vi "Check Rectangles Changed.vi"(8 "error in (no error)":errorcluster, 10 "New Tool":refnum<class "Tool Data.lvclass">, 11 "Tool Data in":refnum<class "Tool Data.lvclass">) -> (0 "error out":errorcluster, 2 "Changed":cluster{bool, "index of element":i32}[](array[cluster]), 3 "Tool Data out":refnum<class "Tool Data.lvclass">)   [LabVIEW 2019, in "Tool Data.lvclass"]
uses:
  Tool Data.lvclass
  Typedefs/Tool Data.Check Changes.ctl
  Parse/Rectangle/Rectangle.lvclass
  Parse/CSSProperties/CSSProperties.lvclass
  Parse/Transform.Matrix/Transform.Matrix.lvclass
  Settings/Rectangle Settings/Rectangle Settings.lvclass
  C:/Users/Albro/Documents/GitHub/AFM-Lithography/lvsrc/Classes/Settings/ObjectSettings/ObjectSettings.lvclass
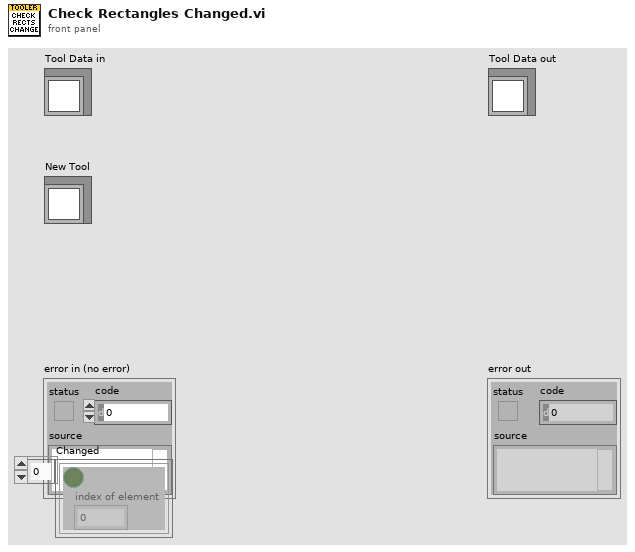
[diagram p1: front panel]
types:
  T1 = typedef "Tool Data.Check Changes.ctl" = cluster{"Data":variant[], "Settings":variant[], "Names":string[]}
  T2 = typedef "Setting Database.lvclass/PublicEvents--Setting Database.RectanglesUpdated.ctl" = refnum<class "Rectangle Settings.lvclass">[]
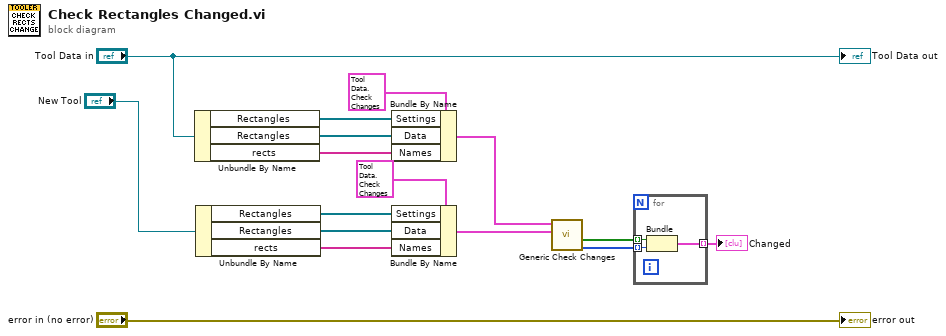
[diagram p0: block diagram]
diagram:
  n1 = Unbundle By Name("Tool Data in") -> ("Rectangles"=w14:T2, "Rectangles"=w13:refnum<class "Rectangle.lvclass">[], "rects"=w12:string[])
  n2 = Unbundle By Name("New Tool") -> ("Rectangles"=w4:T2, "Rectangles"=w5:refnum<class "Rectangle.lvclass">[], "rects"=w10:string[])
  n3 = Bundle By Name(cluster=T1 {"Data"=[variant(refnum<class "Rectangle.lvclass"> refnum), variant(refnum<class "Rectangle.lvclass"> refnum)], "Settings"=[variant(refnum<class "Rectangle Settings.lvclass"> refnum), variant(refnum<class "Rectangle Settings.lvclass"> refnum)], "Names"=["rect14", "rect14-8"]} ("Existing"), "Settings"=w14, "Data"=w13, "Names"=w12) -> (w8:T1)
  n4 = Bundle By Name(cluster=T1 {"Data"=[variant(refnum<class "Rectangle.lvclass"> refnum), variant(refnum<class "Rectangle.lvclass"> refnum)], "Settings"=[variant(refnum<class "Rectangle Settings.lvclass"> refnum), variant(refnum<class "Rectangle Settings.lvclass"> refnum)], "Names"=["rect14", "rect14-8"]} ("Existing"), "Settings"=w4, "Data"=w5, "Names"=w10) -> (w9:T1)
  n5 = call "Generic Check Changes.vi"("New"=w9, "Existing"=w8) -> ("Old Indices"=w6:i32[], "Changed?"=w7:bool[])  [unwired: 6 in, 2 out]
  n6 = for {
    tunnel: w7 -> [w19] mode=indexing
    tunnel: w6 -> [w18] mode=indexing
    tunnel: [w17] -> w3 mode=indexing
    n7 = Bundle(w19, "index of element"=w18) -> (w17:cluster{bool, "index of element":i32})  [unwired: 1 in]
  }
  "Changed" <- w3
  "error out" <- "error in (no error)"
  "Tool Data out" <- "Tool Data in"
